vi "StopEqualization.vi"(8 "error in (no error)":errorcluster, 11 "reference in":refnum<class "sim_MmW.lvclass">) -> (0 "error out":errorcluster, 3 "reference out":refnum<class "sim_MmW.lvclass">)   [LabVIEW 2019, in "sim_MmW.lvclass"]
doc: "Stops calibration procedure"
uses:
  sim_MmW.lvclass
  C:/Barkhausen mmWave radar/Development/LV/Barkhausen mmWave hardware control/Host/SubVIs/mmWave instrument_class/mmWave instrument.lvclass
  mmWave instrument_class/Instrument state.ctl
  mmWave instrument_class/mmWave instrument.lvclass
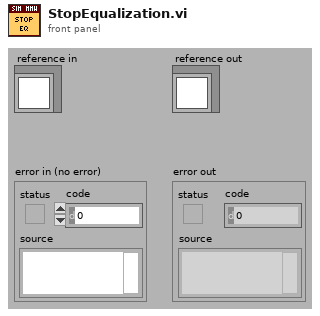
[diagram p1: front panel]
types:
  T1 = typedef "mmWave instrument.lvclass/Instrument state.ctl" = enum16{"Off", "Initialization", "Configuration", "Running", "Calibration"}
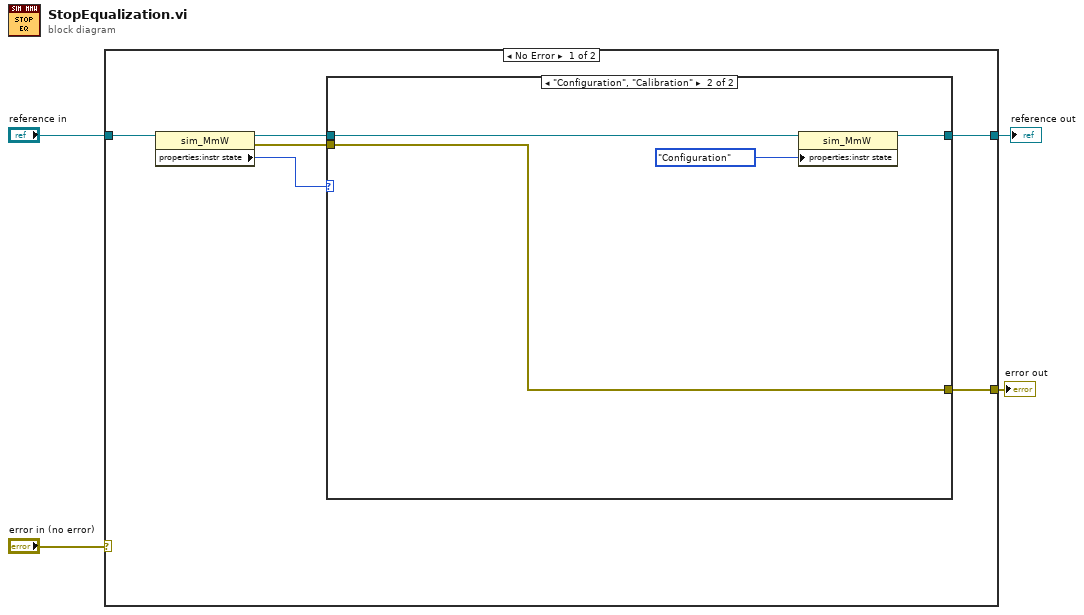
[diagram p0: block diagram]
diagram:
  n1 = case shown="No Error" "error in (no error)" {
    selector: "error in (no error)" -> [_ w18]
    tunnel: [w10 w18] -> w3
    tunnel: [w8 w17] -> w1
    tunnel: "reference in" -> [w9 w17]
    frame No Error {
      n2 = property class="sim_MmW"(reference=w9) -> (reference out=w7:refnum<class "sim_MmW.lvclass">, error out=w6:errorcluster, "properties:instr state"=w5:T1)  [unwired: 1 in]
      n3 = case shown="\"Configuration\", \"Calibration\"" w5 {
        tunnel: [w11 w15] -> w10
        tunnel: [w12 w14] -> w8
        tunnel: w7 -> [w12 w16]
        tunnel: w6 -> [w11 w15]
        frame "Off", Default {
        }
        frame "Configuration", "Calibration" {
          n4 = property class="sim_MmW"(reference=w16, "properties:instr state"=Instrument_state."Configuration" ("instr state")) -> (reference out=w14:refnum<class "sim_MmW.lvclass">)  [unwired: 1 in, 1 out]
        }
      }
    }
    frame Error {
    }
  }
  "error out" <- w3
  "reference out" <- w1
